vi "stop_motor.vi"(10 "Port (All Ports)":T1 items=["Port A"=0, "Port B"=1, "Port C"=2, "Ports A & B"=4, "Ports A & C"=5, "Ports B & C"=6, "All Ports"=3], 11 "停止":bool) -> ()   [LabVIEW 2016, in "main.lvrbt"]
uses:
  main.lvrbt
  <vilib>/NXT/Subs/MotorOutput.ctl
  <vilib>/NXT/Block Support/NXT_OutputPort.ctl
  <vilib>/NXT/Dual Mode Library/Motors/ResetMotor.vi
  <vilib>/NXT/Dual Mode Library/Motors/Rotation.vi
  <vilib>/NXT/Dual Mode Library/Motors/MotorOn.vi
  <vilib>/NXT/Dual Mode Library/Motors/MotorBrake.vi
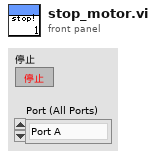
[diagram p1: front panel]
types:
  T1 = typedef "MotorOutput.ctl" = u8
  T2 = typedef "LVHSConnector.ctl" = refnum<class "BrickReference.lvclass">
  T3 = typedef "NXT_OutputPort.ctl" = u8
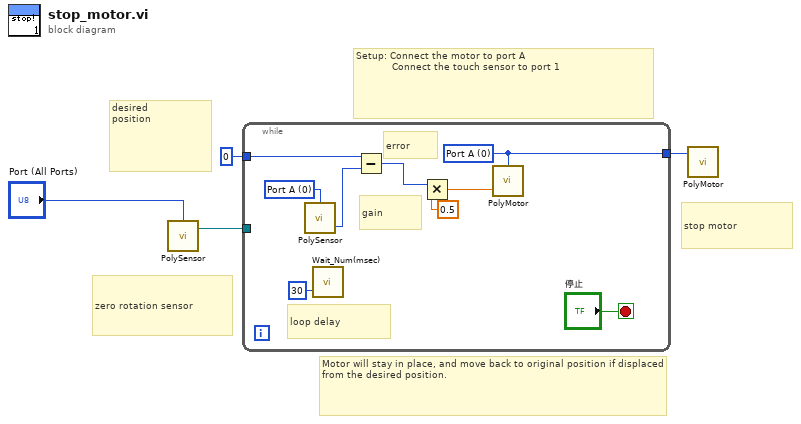
[diagram p0: block diagram]
diagram:
  # "Setup: Connect the motor to port A\n            Connect the touch sensor to port 1"
  # "zero rotation sensor"
  # "desired\nposition"
  # "stop motor"
  # "Motor will stay in place, and move back to original position if displaced from the desired position."
  n1 = call-poly <vilib>:"PolySensor.vi"("Port (All Ports)"="Port (All Ports)") -> ("NXT/EV3"=w2:T2)  [unwired: 1 in, 2 out]
  n2 = while {
    tunnel: 0 ("RotationCount") -> [w11]
    tunnel: [w9] -> w3
    tunnel: w2 -> [_]
    stop <- "停止" stop-if-true
    w6 = T3 0 items=["Port A", "Port B", "Port C", "Port D"] ("Port (Port A)")
    w9 = T1 0 items=["Port A"=0, "Port B"=1, "Port C"=2, "Ports A & B"=4, "Ports A & C"=5, "Ports B & C"=6, "All Ports"=3] ("Output Port (All Ports)")
    # "gain"
    # "error"
    # "loop delay"
    n3 = call-poly <vilib>:"PolySensor.vi"("Port (Port A)"=w6) -> ("Angle of Rotation"=w7:i32)  [unwired: 1 in, 2 out]
    n4 = call <vilib>:"Wait_Num(msec).vi"("Time (100 msec)"=u32 30 ("milliseconds to wait")) -> ()  [unwired: 3 in, 1 out]
    n5 = Subtract(x=w11, y=w7) -> (x-y=w13:i32)
    n6 = Multiply(x=w13, y=sgl 0.5) -> (x*y=w10:sgl)
    n7 = call-poly <vilib>:"PolyMotor.vi"("Power (75)"=w10, "Output Port (All Ports)"=w9) -> ()  [unwired: 1 in, 2 out]
  }
  n8 = call-poly <vilib>:"PolyMotor.vi"("Port (All Ports)"=w3) -> ()  [unwired: 1 in, 3 out]
